vi "RumbleControl.vi"(11 "JoystickDevRef":T1) -> ()   [LabVIEW 2016]
uses:
  <vilib>/Rock Robotics/WPI/Joystick/WPI_JoystickDevRef.ctl
  <vilib>/Rock Robotics/WPI/Joystick/WPI_JoystickDeviceEnum.ctl
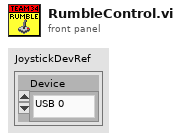
[diagram p1: front panel]
types:
  T1 = typedef "WPI_JoystickDevRef.ctl" = cluster{"Device":T2}
  T2 = typedef "WPI_JoystickDeviceEnum.ctl" = enum16{"USB 0", "USB 1", "USB 2", "USB 3", "USB 4", "USB 5"}
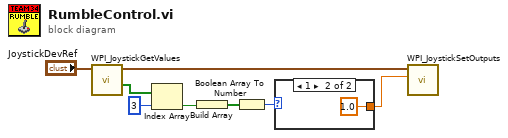
[diagram p0: block diagram]
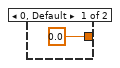
[diagram p2: hidden frame]
diagram:
  n1 = call <vilib>:"WPI_JoystickGetValues.vi"("JoystickDevRef"="JoystickDevRef") -> ("Buttons"=w6:bool[], "JoystickDevRef"=w7:T1)  [unwired: 6 in, 3 out]
  n2 = Index Array(array=w6, index=3) -> (element=w4:bool)
  n3 = Build Array(w4) -> (w3:bool[])
  n4 = Boolean Array To Number(Boolean array=w3) -> (number=w2:u32)
  n5 = case shown="1" w2 {
    tunnel: [sgl 0.0 ("Left Rumble") sgl 1.0 ("Left Rumble")] -> w1
    frame 0, Default {
    }
    frame 1 {
    }
  }
  n6 = call <vilib>:"WPI_JoystickSetOutputs.vi"("Left Rumble"=w1, "JoystickDevRef"=w7) -> ()  [unwired: 8 in, 2 out]
